vi "USRP Dummy DMA to Memory (Host).vi"() -> ()   [LabVIEW 2016]
uses:
  <vilib>/rvi/interface/nirviMethod/nirviMethod.xnode
  <vilib>/rvi/errors/niLvFpgaMergeErrorWithErrorCode.vi
  <vilib>/rvi/interface/nirviReadWriteControl/nirviReadWriteControl.xnode
  <vilib>/rvi/interface/Simulation/niFpgaSimulationCallBeginRW.vi
  <vilib>/rvi/errors/niLvFpgaAdjustHostInterfaceError.vi
  <instrlib>/niUsrpRio/Config/v1/Host/niUsrpRio Config v1 Host.lvlib
  <vilib>/rvi/interface/nirviOpenFPGA/nirviOpenFPGA.xnode
  <vilib>/rvi/interface/nirviCloseFPGA/nirviCloseFPGA.xnode
  NiFpgaLv.dll
  <vilib>/Utility/error.llb/Error Cluster From Error Code.vi
  <vilib>/FPGAPlugInAG/Dynamic/niLvFpga_Download_Dynamic.vi
  <vilib>/FPGAPlugInAG/Dynamic/niLvFpga_Run_Dynamic.vi
  FPGA Bitfiles/USRP-RIO-Streami_DummyDMA_USRPDummy(FPGA)_kay5ptBR-r4.lvbitx
  <vilib>/FPGAPlugInAG/USRP 294xR; 295xR 200 MSps/niLvFpga_Open_USRP 294xR; 295xR 200 MSps.vi
  <vilib>/rvi/interface/common/dynamic/niFpgaDynamicAddResources.vi
  <vilib>/FPGAPlugInAG/Dynamic/niLvFpga_StopFifo_Dynamic.vi
  <vilib>/FPGAPlugInAG/Dynamic/niLvFpga_ConfigureFifo_Dynamic.vi
  <vilib>/FPGAPlugInAG/Dynamic/niLvFpga_StartFifo_Dynamic.vi
  <vilib>/FPGAPlugInAG/Dynamic/niLvFpga_ReadFifo_Dynamic.vi
  <vilib>/FPGAPlugInAG/Dynamic/niLvFpga_Close_Dynamic.vi
  <vilib>/userdefined/High Color/nirio_resource_hc.ctl
panel:
  in  "Fixed Fetch?":bool=TRUE
  out "Random Number":u64 format="%016x"
  in  "Decimate (200MHz)":u32=2
  out "Host Transfer Slider":u64(slide) scale=0.0..68719476736.0
  in  "Flush FIFO?":bool
  out "Control Loop":i32
  in  "Host FIFO Fetch":u32=131072
  in  "Reset Host Count?":bool
  in  "Stop Transfer?":bool
  in  "Reset FPGA Count?":bool
  out "FPGA Side FIFO":cluster{u32, u32}(slide)={66, 63} scale=0.0..2047.0
  out "Host Side FIFO":cluster{u32, u32}(slide) scale=0.0..67108863.0
  out "Data Loop":i32
  out "Fetch Loop":i32
  out "Host Count":u64
  in  "Number of Samples":u64=68719476736
  out "FPGA Count":u64
  in  "Start Transfer":bool
  in  "terminate":bool
  out "Elements Remaining":u32
  out "Data":u64[](array[numeric]) format="%016x"
  out "Timeout Counts":u64
  in  "Reset Timeouts?":bool
  out "Actual Depth":u32
  in  "Host Requested Depth":u32=67108864
  out "error out":errorcluster
  in  "error in (no error)":errorcluster
  in  "Resource Name":T1="PXI2Slot18Port1Dev1"
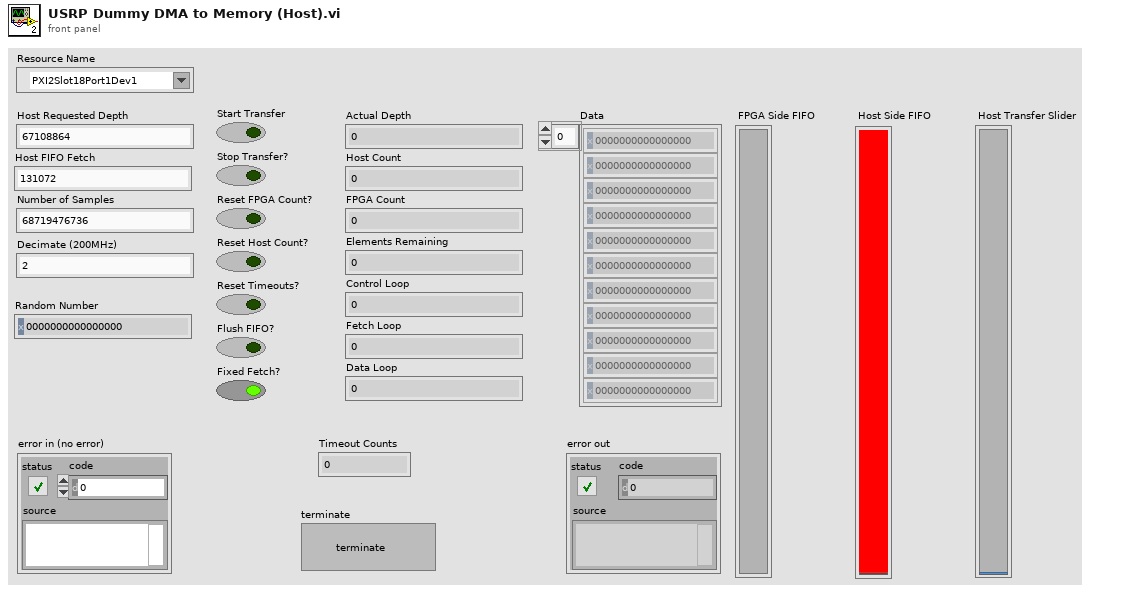
[diagram p1: front panel]
types:
  T1 = typedef "nirio_resource_hc.ctl" = tag
  T2 = typedef "niUsrpRio Config v1 Host.lvlib/niUsrpRio Session.ctl" = cluster{"FPGA Interface":refnum<k20>, "RIO Interface Number":u32, "Data Clock Rate":u32, "FPGA Data Clock Rate":u32, "Global Settings Register Bus":T3, "Radio 0 Settings Register Bus":T3, "Radio 1 Settings Register Bus":T3, "Radio Settings Bus Semaphore":T4, "DB Queues":T5[], "Characterization Data Valid?":bool, "EEPROM Header":T6, "Device Data Header":T7, "EEPROM Characterization Header":T8, "Characterization Data":T9[], "FPGA Current Version":u32, "FPGA Oldest Compatible Version":u32, "Fixed Logic Current Version":u32, "Fixed Logic Oldest Compatible Version":u32, "FPGA Radio Settings Bus Current Version":u32, "FPGA Radio Settings Bus Oldest Compatible Version":u32, "FPGA Board Config Current Version":u32, "FPGA Board Config Oldest Compatible Version":u32, "Daughterboard Clock Rate":u32, "daughterboard configuration session handles":u64[]}
  T3 = typedef "niInstr Register Bus v0 Host.lvlib/Register Bus Session.ctl" = refnum<queue>
  T4 = typedef "Semaphore RefNum" = refnum<k1>
  T5 = typedef "niUsrpRio Config v1 Host.lvlib/DB Queue Reference.ctl" = refnum<queue>
  T6 = typedef "niUsrpRio Config v1 Host.lvlib/EEPROM Header.ctl" = cluster{"Checksum":u32, "Product Code":u16, "Hardware Current Version":u16, "Hardware Oldest Compatible Version":u16, "EEPROM Map Current Version":u16, "EEPROM Map Oldest Compatible Version":u16, "User Password":string, "Pointer to Factory Header":u32, "Pointer to User Header":u32, "Recommended Interval":u16, "Number of Reserved Bytes":i32, "Number of Daughterboards":u8, "Daughterboard IDs":u16[], "Daughterboard Serial Numbers":string[]}
  T7 = typedef "niUsrpRio Config v1 Host.lvlib/EEPROM Device Data Header.ctl" = cluster{"Checksum":u32, "Number of Channels":u8, "Number of Gain Settings":u16[], "Pointer to Characterization Data":u32[], "Number of Reserved Bytes":i32, "Number of Frequencies":u16[]}
  T8 = typedef "niUsrpRio Config v1 Host.lvlib/EEPROM Characterization Header.ctl" = cluster{"Checksum":u32, "Date":timestamp, "Temperature":sgl, "Misc. Info":string, "Pointer to Device Data Header":u32, "Number of Reserved Bytes":i32}
  T9 = typedef "niUsrpRio Config v1 Host.lvlib/Characterization Data.ctl" = cluster{"Gains[dB]":dbl[], "Frequencies [Hz]":dbl[], "IQ Imbalance Table":T10[], "Measured Gains[dB]":dbl[][]}
  T10 = typedef "niUsrpRio Config v1 Host.lvlib/IQ Imbalance.ctl" = cluster{"Gain Imbalance [linear]":dbl, "Phase Imbalance [radians]":dbl, "Offset":cdb}
  T11 = cluster{"Maximum Amount Used":u32, "Current Amount Used":u32}
  T12 = cluster{"Running Max":u32, "Elements Remaining":u32}
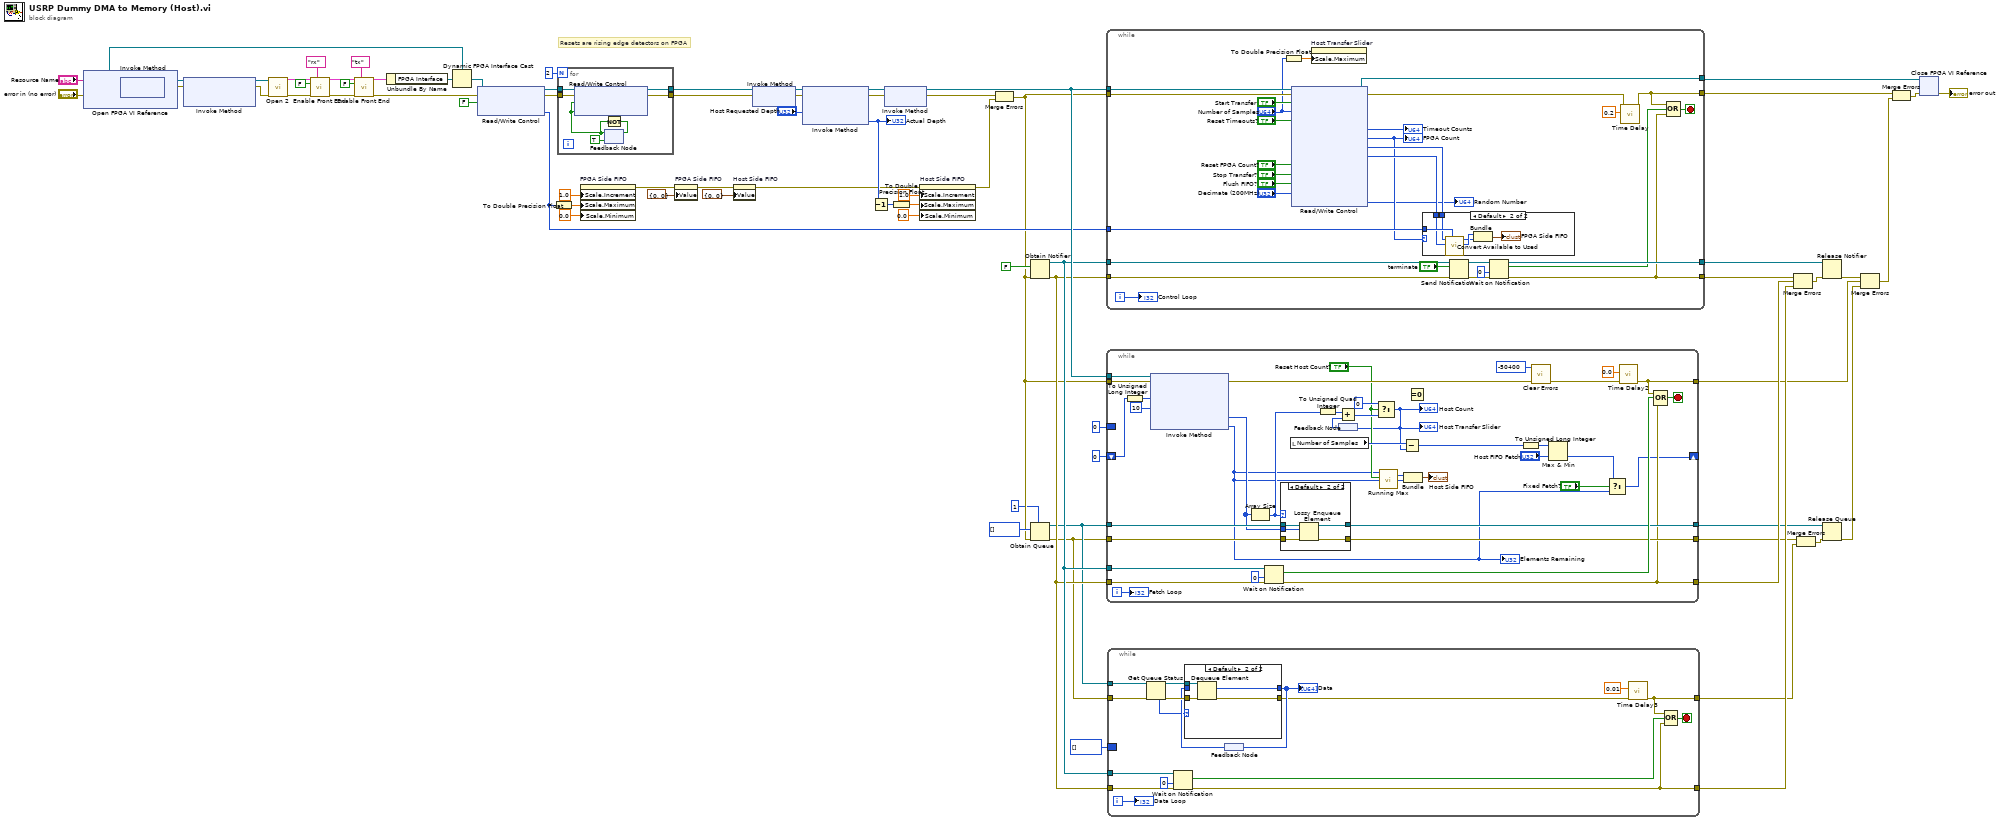
[diagram p0: block diagram]
diagram:
  # "Resets are rising edge detectors on FPGA"
  n1 = xnode "Open FPGA VI Reference"("error in"="error in (no error)", "resource name"="Resource Name") -> ("FPGA VI Reference Out"=w7:refnum<k20>, "error out"=w6:errorcluster)
  n2 = xnode "Invoke Method"("FPGA VI Reference In"=w7, "error in"=w6) -> ("FPGA VI Reference Out"=w5:refnum<k20>, "error out"=w4:errorcluster)
  n3 = xnode "Invoke Method"("FPGA VI Reference In"=w5, "error in"=w4) -> ("FPGA VI Reference Out"=w3:refnum<k20>, "error out"=w2:errorcluster)  [unwired: 1 in]
  n4 = call <instrlib>:"Open 2.vi"("fpga ref"=w3, "error in"=w2) -> ("niUsrpRio Session (out)"=w65:T2, "error out"=w70:errorcluster)  [unwired: 12 in]
  n5 = call <instrlib>:"Enable Front End.vi"("niUsrpRio Session"=w65, "scope"="rx", "enable"=FALSE, "error in"=w70) -> ("niUsrpRio Session (out)"=w66:T2, "error out"=w69:errorcluster)  [unwired: 10 in]
  n6 = call <instrlib>:"Enable Front End.vi"("niUsrpRio Session"=w66, "scope"="tx", "enable"=FALSE, "error in"=w69) -> ("niUsrpRio Session (out)"=w62:T2, "error out"=w61:errorcluster)  [unwired: 10 in]
  n7 = Unbundle By Name(w62) -> ("FPGA Interface"=w60:refnum<k20>)
  n8 = Dynamic FPGA Interface Cast(Session In=w7, Type=w60) -> (Session Out=w59:refnum<k20>)
  n9 = xnode "Read/Write Control"("FPGA VI Reference In"=w59, "error in"=w61, "Start Transfer?"=FALSE ("send data?")) -> ("FPGA VI Reference Out"=w36:refnum<k20>, "error out"=w35:errorcluster, "FPGA FIFO Depth"=w21:u32)
  n10 = To Double Precision Float(number=w21) -> (double precision float=w23:dbl)
  n11 = for {
    N: 2 -> [_]
    tunnel: w36 -> [w83]
    tunnel: w35 -> [w82]
    tunnel: [w81] -> w34
    tunnel: [w80] -> w33
    n12 = feedback #1(TRUE) -> (w78:bool)
    n13 = xnode "Read/Write Control"("FPGA VI Reference In"=w83, "error in"=w82, "Reset Timeouts?"=w78, "Reset FPGA Count?"=w78) -> ("FPGA VI Reference Out"=w81:refnum<k20>, "error out"=w80:errorcluster)
    n14 = Not(x=w78) -> (.not. x?=w77:bool)
    n15 = feedback-in #1(w77) -> ()
  }
  n16 = property on="FPGA Side FIFO" class="Slide (strict)"("Scale.Increment"=1.0 ("Scale.Range:Increment"), "Scale.Maximum"=w23, "Scale.Minimum"=0.0 ("Scale.Range:Minimum")) -> (error out=w16:errorcluster)  [unwired: 2 in, 1 out]
  n17 = property on="FPGA Side FIFO" class="Slide (strict)"(error in=w16, "Value"=cluster{u32, u32} {0, 0} ("FPGA Side FIFO")) -> (error out=w19:errorcluster)  [unwired: 1 in, 1 out]
  n18 = property on="Host Side FIFO" class="Slide (strict)"(error in=w19, "Value"=cluster{u32, u32} {0, 0} ("FPGA Side FIFO")) -> (error out=w15:errorcluster)  [unwired: 1 in, 1 out]
  n19 = xnode "Invoke Method"("FPGA VI Reference In"=w34, "error in"=w33) -> ("FPGA VI Reference Out"=w76:refnum<k20>, "error out"=w75:errorcluster)
  n20 = xnode "Invoke Method"("FPGA VI Reference In"=w76, "error in"=w75, "Requested Depth"="Host Requested Depth") -> ("FPGA VI Reference Out"=w72:refnum<k20>, "error out"=w73:errorcluster, "Actual Depth"=w20:u32)
  "Actual Depth" <- w20
  n21 = Decrement(x=w20) -> (x-1=w26:u32)
  n22 = xnode "Invoke Method"("FPGA VI Reference In"=w72, "error in"=w73) -> ("FPGA VI Reference Out"=w56:refnum<k20>, "error out"=w22:errorcluster)
  n23 = To Double Precision Float(number=w26) -> (double precision float=w8:dbl)
  n24 = property on="Host Side FIFO" class="Slide (strict)"(error in=w15, "Scale.Increment"=1.0 ("Data Entry Limits:Increment"), "Scale.Maximum"=w8, "Scale.Minimum"=0.0 ("Data Entry Limits:Minimum")) -> (error out=w13:errorcluster)  [unwired: 1 in, 1 out]
  n25 = Merge Errors(w22, w13) -> (w14:errorcluster)
  n26 = Obtain Notifier(notification data type=FALSE, error in (no error)=w14) -> (notifier out=w48:refnum<notifier>, error out=w47:errorcluster)  [unwired: 2 in, 1 out]
  n27 = Obtain Queue(max queue size (-1, unlimited)=1, element data type=u64[] [] ("Data"), error in (no error)=w14) -> (queue out=w40:refnum<queue>, error out=w39:errorcluster)  [unwired: 2 in, 1 out]
  n28 = while {
    tunnel: w56 -> [w114]
    tunnel: w14 -> [w113]
    tunnel: w48 -> [w110]
    tunnel: w47 -> [w109]
    tunnel: [w104] -> w53
    tunnel: [w97] -> w52
    tunnel: [w99] -> w31
    tunnel: [w98] -> w30
    tunnel: w21 -> [w96]
    i -> [w89]
    stop <- w103 stop-if-true
    n29 = To Double Precision Float(number="Number of Samples") -> (double precision float=w86:dbl)
    n30 = xnode "Read/Write Control"("FPGA VI Reference In"=w114, "error in"=w113, "Start Transfer?"="Start Transfer", "Number of Samples"="Number of Samples", "Reset Timeouts?"="Reset Timeouts?", "Reset FPGA Count?"="Reset FPGA Count?", "Stop Transfer?"="Stop Transfer?", "Flush FIFO?"="Flush FIFO?", "Decimate (200MHz)"="Decimate (200MHz)") -> ("FPGA VI Reference Out"=w98:refnum<k20>, "error out"=w112:errorcluster, "Timeout Count"=→"Timeout Counts":u64, "FPGA Count"=w90:u64, "Space Available"=w95:u32, "Min Space Available"=w93:u32, "Random Number"=→"Random Number":u64)
    "FPGA Count" <- w90
    n31 = property on="Host Transfer Slider" class="Slide (strict)"("Scale.Maximum"=w86) -> ()  [unwired: 2 in, 2 out]
    n32 = case shown="Default" w90 {
      tunnel: w96 -> [_ w120]
      tunnel: w95 -> [_ w119]
      tunnel: w93 -> [_ w118]
      frame 0 {
      }
      frame Default {
        n33 = call "Convert Available to Used.vi"("Size"=w120, "Minimum Amount Available"=w118, "Current Amount Available"=w119) -> ("Maximum Amount Used"=w117:u32, "Current Amount Used"=w116:u32)  [unwired: 5 in]
        n34 = Bundle("Maximum Amount Used"=w117, "Current Amount Used"=w116) -> (→"FPGA Side FIFO":T11)  [unwired: 1 in]
      }
    }
    n35 = Send Notification(notification="terminate", notifier=w110, error in (no error)=w109) -> (notifier out=w106:refnum<notifier>, error out=w105:errorcluster)
    n36 = Wait on Notification(notifier=w106, timeout in ms (-1)=0, error in (no error)=w105) -> (notifier out=w104:refnum<notifier>, notification=w102:bool, error out=w97:errorcluster)  [unwired: 1 in, 1 out]
    n37 = call "Time Delay"("error in (no error)"=w112, "Delay Time (s)"=0.2) -> ("error out"=w99:errorcluster)  [unwired: 9 in]
    n38 = Compound Arithmetic op=OR(w99, w102, w97) -> (w103:bool)
    "Control Loop" <- w89
  }
  n39 = while {
    tunnel: [w154] -> w32
    tunnel: w56 -> [w157]
    tunnel: w14 -> [w156]
    border: u64 0 -> [_]
    tunnel: w48 -> [w150]
    tunnel: w47 -> [w149]
    tunnel: [w140] -> w50
    tunnel: [w145] -> w44
    tunnel: w40 -> [w146]
    tunnel: w39 -> [w144]
    tunnel: [w143] -> w43
    shift-right: [w126] -> _
    shift-left: u64 0 -> [w134]
    i -> [w147]
    stop <- w152 stop-if-true
    n40 = To Unsigned Long Integer(number=w134) -> (unsigned 32bit integer=w133:u32)
    n41 = xnode "Invoke Method"("FPGA VI Reference In"=w157, "error in"=w156, "Number of Elements"=w133, "Timeout (ms)"=10) -> ("error out"=w142:errorcluster, "Data"=w141:u64[], "Elements Remaining"=w125:u32)  [unwired: 1 out]
    "Elements Remaining" <- w125
    n42 = Array Size(array=w141) -> (size(s)=w137:i32)
    n43 = Wait on Notification(notifier=w150, timeout in ms (-1)=0, error in (no error)=w149) -> (notification=w148:bool, error out=w140:errorcluster)  [unwired: 1 in, 2 out]
    n44 = case shown="Default" w137 {
      tunnel: w146 -> [w161 w166]
      tunnel: [w161 w165] -> w145
      tunnel: w144 -> [w160 w164]
      tunnel: [w160 w163] -> w143
      tunnel: w141 -> [_ w162]
      frame 0 {
      }
      frame Default {
        n45 = Lossy Enqueue Element(queue=w166, element=w162, error in (no error)=w164) -> (queue out=w165:refnum<queue>, error out=w163:errorcluster)  [unwired: 2 out]
      }
    }
    n46 = local read "Number of Samples"() -> (w136:u64)
    n47 = To Unsigned Quad Integer(1:w137) -> (0:w159:u64)
    n48 = feedback #2() -> (w158:u64)
    n49 = Add(x=w159, y=w158) -> (x+y=w139:u64)
    n50 = Select(t=u64 0, s="Reset Host Count?", f=w139) -> (s? t:f=w123:u64)
    "Host Count" <- w123
    "Host Transfer Slider" <- w123
    n51 = feedback-in #2(w123) -> ()
    n52 = call "Running Max.vi"("Reset"="Reset Host Count?", "Next Value"=w125) -> ("Running Max"=w130:u32)  [unwired: 5 in]
    n53 = Subtract(x=w136, y=w123) -> (x-y=w135:u64)
    n54 = Bundle("Running Max"=w130, "Elements Remaining"=w125) -> (→"Host Side FIFO":T12)  [unwired: 1 in]
    n55 = Equal To 0?() -> ()  [unwired: 1 in, 1 out]
    n56 = To Unsigned Long Integer(number=w135) -> (unsigned 32bit integer=w124:u32)
    n57 = call <vilib>:"Clear Errors.vi"("error in (no error)"=w142, "specific error code to clear (0: all)"=-50400) -> ("error out"=w132:errorcluster)  [unwired: 4 in, 1 out]
    n58 = Max & Min(x=w124, y="Host FIFO Fetch") -> (min(x,y)=w121:u32)  [unwired: 1 out]
    n59 = Select(t=w121, s="Fixed Fetch?", f=w125) -> (s? t:f=w126:u32)
    n60 = call "Time Delay2"("error in (no error)"=w132, "Delay Time (s)"=0.0) -> ("error out"=w154:errorcluster)  [unwired: 9 in]
    n61 = Compound Arithmetic op=OR(w154, w148, w140) -> (w152:bool)
    "Fetch Loop" <- w147
  }
  n62 = while {
    tunnel: w48 -> [w181]
    tunnel: w47 -> [w180]
    tunnel: [w167] -> w46
    tunnel: w40 -> [w178]
    tunnel: w39 -> [w177]
    tunnel: [w169] -> w38
    border: u64[] [] -> [_]
    i -> [w183]
    stop <- w171 stop-if-true
    n63 = Get Queue Status(queue=w178, error in (no error)=w177) -> (queue out=w175:refnum<queue>, error out=w176:errorcluster, # elements in queue=w172:i32)  [unwired: 1 in, 5 out]
    n64 = Wait on Notification(notifier=w181, timeout in ms (-1)=0, error in (no error)=w180) -> (notification=w179:bool, error out=w167:errorcluster)  [unwired: 1 in, 2 out]
    n65 = feedback #3() -> (w174:u64[])
    n66 = case shown="Default" w172 {
      tunnel: [w185 w189] -> w170
      tunnel: [w184 w186] -> w173
      tunnel: w176 -> [w185 w188]
      tunnel: w175 -> [_ w187]
      tunnel: w174 -> [w184 _]
      frame 0 {
      }
      frame Default {
        n67 = Dequeue Element(queue=w187, error in (no error)=w188) -> (element=w186:u64[], error out=w189:errorcluster)  [unwired: 1 in, 2 out]
      }
    }
    "Data" <- w173
    n68 = feedback-in #3(w173) -> ()
    n69 = call "Time Delay3"("error in (no error)"=w170, "Delay Time (s)"=0.01) -> ("error out"=w169:errorcluster)  [unwired: 9 in]
    n70 = Compound Arithmetic op=OR(w169, w179, w167) -> (w171:bool)
    "Data Loop" <- w183
  }
  n71 = Merge Errors(w52, w50, w46) -> (w51:errorcluster)
  n72 = Merge Errors(w43, w38) -> (w42:errorcluster)
  n73 = Release Notifier(notifier=w53, error in (no error)=w51) -> (error out=w49:errorcluster)  [unwired: 1 in, 2 out]
  n74 = Release Queue(queue=w44, error in (no error)=w42) -> (error out=w41:errorcluster)  [unwired: 1 in, 2 out]
  n75 = Merge Errors(w49, w32, w41) -> (w9:errorcluster)
  n76 = Merge Errors(w31, w9) -> (w10:errorcluster)
  n77 = xnode "Close FPGA VI Reference"("FPGA VI Reference In"=w30, "error in"=w10) -> ("error out"=→"error out":errorcluster)
